vi "Main_VI.vi"(7 "ChannelList":string, 8 "error in (no error)":errorcluster {"code" format="%.0x"}, 9 "Range":dbl, 10 "Combo Box":string(combo), 11 "resource string":string="USB0::0x2A8D::0x5101::MY58039196::INSTR") -> (0 "error out":errorcluster)   [LabVIEW 2021]
uses:
  <instrlib>/Keysight DAQ970/Keysight DAQ970.lvlib
panel:
  out "Val":dbl[][](array[numeric])
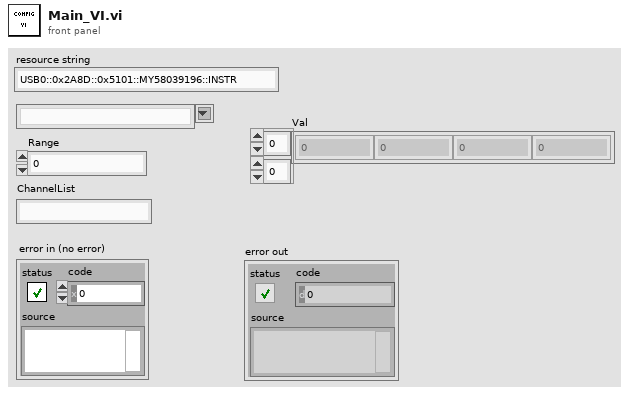
[diagram p1: front panel]
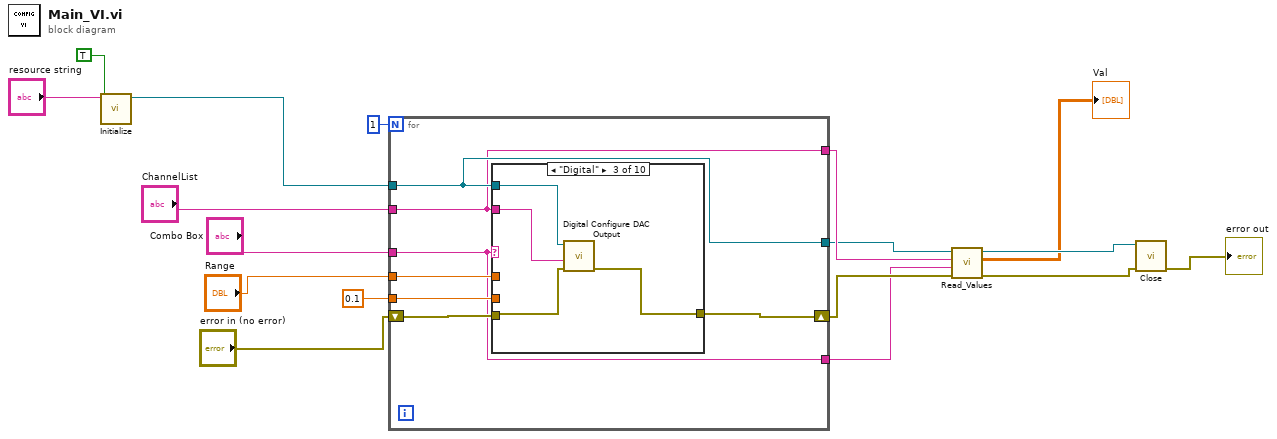
[diagram p0: block diagram]
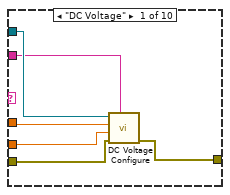
[diagram p2: hidden frame]
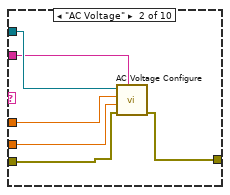
[diagram p3: hidden frame]
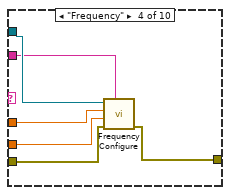
[diagram p4: hidden frame]
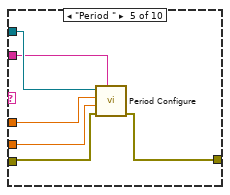
[diagram p5: hidden frame]
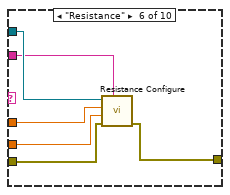
[diagram p6: hidden frame]
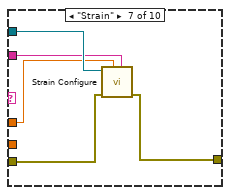
[diagram p7: hidden frame]
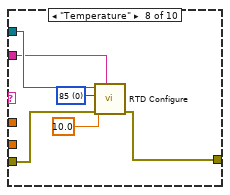
[diagram p8: hidden frame]
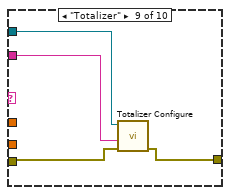
[diagram p9: hidden frame]
diagram:
  n1 = call <instrlib>:"Initialize.vi"("id query (Off)"=TRUE, "resource string"="resource string") -> ("instrument handle out"=w13:refnum<k15>)  [unwired: 8 in, 1 out]
  n2 = for {
    N: 1 -> [_]
    shift-right: [w24] -> w9
    shift-left: "error in (no error)" -> [w23]
    tunnel: "Combo Box" -> [w19]
    tunnel: "ChannelList" -> [w18]
    tunnel: "Range" -> [w22]
    tunnel: w13 -> [w21]
    tunnel: [w21] -> w4
    tunnel: 0.1 ("Resolution") -> [w20]
    tunnel: [w19] -> w5
    tunnel: [w18] -> w6
    n3 = case shown="\"Digital\"" w19 {
      tunnel: [w27 w32 w37 w42 w48 w54 w59 w65 w70 w74] -> w24
      tunnel: w23 -> [w28 w33 w38 w43 w49 w55 w60 w66 w71 w74]
      tunnel: w18 -> [w29 w35 w39 w45 w51 w57 w62 w68 w72 _]
      tunnel: w22 -> [w26 w34 _ w44 w50 w56 w61 _ _ _]
      tunnel: w21 -> [w30 w36 w40 w46 w52 w58 w63 w69 w73 _]
      tunnel: w20 -> [w25 w31 _ w41 w47 w53 _ _ _ _]
      frame "DC Voltage" {
        n4 = call <instrlib>:"DC Voltage Configure.vi"("ChannelList"=w29, "error in (no error)"=w28, "Resolution"=w25, "Range"=w26, "instrument handle"=w30) -> ("error out"=w27:errorcluster)  [unwired: 5 in, 1 out]
      }
      frame "AC Voltage" {
        n5 = call <instrlib>:"AC Voltage Configure.vi"("ChannelList"=w35, "error in (no error)"=w33, "Resolution"=w31, "Range"=w34, "instrument handle"=w36) -> ("error out"=w32:errorcluster)  [unwired: 5 in, 1 out]
      }
      frame "Digital" {
        n6 = call <instrlib>:"Digital Configure DAC Output.vi"("error in (no error)"=w38, "ChannelList"=w39, "instrument handle"=w40) -> ("error out"=w37:errorcluster)  [unwired: 7 in, 1 out]
      }
      frame "Frequency" {
        n7 = call <instrlib>:"Frequency Configure.vi"("ChannelList"=w45, "error in (no error)"=w43, "Resolution"=w41, "Range"=w44, "instrument handle"=w46) -> ("error out"=w42:errorcluster)  [unwired: 5 in, 1 out]
      }
      frame "Period " {
        n8 = call <instrlib>:"Period Configure.vi"("ChannelList"=w51, "error in (no error)"=w49, "Resolution"=w47, "Range"=w50, "instrument handle"=w52) -> ("error out"=w48:errorcluster)  [unwired: 5 in, 1 out]
      }
      frame "Resistance" {
        n9 = call <instrlib>:"Resistance Configure.vi"("ChannelList"=w57, "error in (no error)"=w55, "Resolution"=w53, "Range"=w56, "instrument handle"=w58) -> ("error out"=w54:errorcluster)  [unwired: 5 in, 1 out]
      }
      frame "Strain" {
        n10 = call <instrlib>:"Strain Configure.vi"("ChannelList"=w62, "Range"=w61, "error in (no error)"=w60, "instrument handle"=w63) -> ("error out"=w59:errorcluster)  [unwired: 6 in, 1 out]
      }
      frame "Temperature" {
        w67 = 0 items=["85", "91"] ("RtdAlpha (85)")
        n11 = call <instrlib>:"RTD Configure.vi"("ChannelList"=w68, "error in (no error)"=w66, "Resolution"=10.0, "RtdAlpha (85)"=w67, "instrument handle"=w69) -> ("error out"=w65:errorcluster)  [unwired: 5 in, 1 out]
      }
      frame "Totalizer" {
        n12 = call <instrlib>:"Totalizer Configure.vi"("error in (no error)"=w71, "ChannelList"=w72, "instrument handle"=w73) -> ("error out"=w70:errorcluster)  [unwired: 7 in, 1 out]
      }
      frame Default {
      }
    }
  }
  n13 = call "Read_Values.vi"("error in (no error)"=w9, "Combo Box"=w5, "ChannelList"=w6, "instrument handle out"=w4) -> ("error out"=w1:errorcluster, "Val"=→"Val":dbl[][], "instrument handle 2"=w8:refnum<k15>)  [unwired: 4 in]
  n14 = call <instrlib>:"Close.vi"("error in (no error)"=w1, "instrument handle"=w8) -> ("error out"=→"error out":errorcluster)  [unwired: 9 in]
